vi "HDF5_Test2.vi"   [LabVIEW 2018]
uses:
  <vilib>/addons/h5labview2/base/H5Equery.vi
  HDF5/lib_path_mod_20200519.vi
  HDF5/HDF5_ToneInfoClust.ctl
  <vilib>/addons/h5labview2/attrib/H5Awrite.llb/H5Awrite.xnode
  <vilib>/addons/h5labview2/base/hid_t_renamed.ctl
  <vilib>/addons/h5labview2/file/H5F.lvlib
  <vilib>/addons/h5labview2/file/H5Fmode.ctl
  Controls/Clusts/LogLoopClust.ctl
  Controls/ToneInfoClust.ctl
  Controls/Clusts/ChannelToneData.ctl
  Controls/Enums/TargetNumber.ctl
  <vilib>/addons/h5labview2/group/H5G.lvlib
  <vilib>/addons/h5labview2/dataset/H5D.lvlib
  HDF5/HDF5_Tone_refs.ctl
  HDF5/HDF5_Complex_Refs.ctl
  HDF5/HDF5_ADAM_Refs.ctl
  HDF5/HDF5_Filter_refs.ctl
  HDF5/HDF5_AI_refs.ctl
  Controls/PathsCluster.ctl
  Controls/Enums/ScaleMeasure.ctl
  Controls/Clusts/FPGA_Scale.ctl
  Controls/Clusts/FreqShift.ctl
  Controls/Clusts/FP_UserTargetConfig.ctl
  Controls/Clusts/FrontPanel_UserConfig.ctl
  Controls/Clusts/UserConfig.ctl
  Controls/Clusts/Config_Clust.ctl
  Controls/Clusts/WeatherRefs.ctl
  HDF5/UPS_refs.ctl
  HDF5/HDF5_Health_Refs.ctl
  HDF5/HDF5_Disdrometer_Refs.ctl
  HDF5/HDF5_Validty_refs.ctl
  HDF5/TC_Tone_refs.ctl
  HDF5/HDF5_Noise_refs.ctl
  Controls/Clusts/ToneGroupRefsClust.ctl
  Controls/Clusts/TimeDomainData.ctl
  HDF5/HDF5_ADAM_Data.ctl
  Controls/Clusts/TE_Data_Clust.ctl
  Controls/Clusts/WeatherDataClust.ctl
  Disdrometer/Disdrometer_Status_Cluster.ctl
  HDF5/DisdromterSummaryData.ctl
  HDF5/DisdrometerData.ctl
  HDF5/HDF5_NoiseInfoClust.ctl
  Controls/Clusts/AI_Clust.ctl
  HDF5/TC_Data_Structure.ctl
  Controls/Clusts/ToneLogBuffered.ctl
  Controls/Clusts/LogDataClust.ctl
  Controls/Clusts/HDF5_File_Refs.ctl
  Controls/RadioButtons/FilterEnableRadio.ctl
  Controls/Clusts/Inclinometer_User_Cfg.ctl
  Controls/Clusts/AlarmThresh_OneChan.ctl
  Controls/Clusts/AlarmSettingsClust.ctl
  Controls/Clusts/ErrorStatus.ctl
  Controls/Clusts/ValidityWeatherClust.ctl
  Controls/Clusts/SaturationMonitorBuffer.ctl
  Controls/Clusts/HDF5_10HzRefs.ctl
  Controls/Clusts/Saturation_Status_Clust.ctl
  <vilib>/addons/h5labview2/base/hid_t.ctl
  Controls/Clusts/DigOutClust.ctl
types:
  T1 = typedef "HDF5_ToneInfoClust.ctl" = cluster{"Timestring":string, "Timestamp":dbl, "MaxValue":dbl, "PeakLoc":dbl, "df":dbl}
  T2 = typedef "LogLoopClust.ctl" = cluster{"base path":path, "PathNow1":path, "PathNow2":path, "DateNow":string, "NAS path":path, "LogFiltStage":bool, "Config":T3, "HDFRefs1":T14, "HDFRefs2":T14, "LogData":T29, "AlarmCfg":T43, "DO":bool[], "AllAlarms":T45[], "Alarm Status":T46, "SaturationStatus":T47, "WeatherStatus":bool[], "10HzRefs":T48}
  T3 = typedef "Config_Clust.ctl" = cluster{"UsrCfg":T4, "FP_User":T6}
  T4 = typedef "UserConfig.ctl" = cluster{"Paths":T5, "SampleRate":dbl}
  T5 = typedef "PathsCluster.ctl" = cluster{"CfgFile":path, "LogFolder":path, "LogFile":path, "NAS path":path, "ThreshFile":path, "RedunFolder":path}
  T6 = typedef "FrontPanel_UserConfig.ctl" = cluster{"#NoiseSums":u32, "Max_df":u32, "AvgAvg":bool, "#Avg":u16, "AutoCenter":bool, "Inclin":T7, "1":T8, "2":T8, "3":T8, "4":T8, "Target to Probe":T13, "SNR_Thresh":dbl, "Paths":T5, "Connex_Location":string, "SimulateFPGA":bool}
  T7 = typedef "Inclinometer_User_Cfg.ctl" = cluster{"Vmin":dbl, "Vmax":dbl, "Angle_min":dbl, "Angle_max":dbl, "Offset":dbl, "Pos_Neg":bool}
  T8 = typedef "FP_UserTargetConfig.ctl" = cluster{"Cal_":T9, "Beac":T9, "Scale":T10, "Offset":fxp<+/-,16,16>, "Scale_Noise":fxp<+/-,30,30>, "Scale_Step1":fxp<+/-,17,17>, "Scale_In_RT":ext, "ScaleMeas":fxp<+/-,16,1>, "FreqsToRemove":i32[], "Width":i32[], "ScaleMeasEnum":T11, "FilterEnab":T12}
  T9 = typedef "FreqShift.ctl" = cluster{"Fine":dbl, "Coarse_":dbl}
  T10 = typedef "FPGA_Scale.ctl" = cluster{"Step4":fxp<+/-,23,23>, "Step5":fxp<+/-,23,23>, "Step6":fxp<+/-,23,23>, "Step7":fxp<+/-,23,23>}
  T11 = typedef "ScaleMeasure.ctl" = enum16{"1", "10", "50", "42"}
  T12 = typedef "FilterEnableRadio.ctl" = enum32{"None", "Step 1", "Frequency Shift", "Step 4", "Step 5", "Step 6", "Step 7"}
  T13 = typedef "TargetNumber.ctl" = enum16{"1", "2", "3", "4"}
  T14 = typedef "HDF5_File_Refs.ctl" = cluster{"File":T15, "ToneRefs":T16[], "NoiseRefs":T18[], "TC_Refs":T19, "ValidRefs":T20, "DisdromRefs":T21, "TE_Refs":T22, "UPS_Refs_Deprecated":T23, "Weath_Refs":T24, "AI_Refs":T25, "Filter_Refs":T26, "ADAM_Refs":T27, "Complex":T28[]}
  T15 = typedef "hid_t.ctl" = i32
  T16 = typedef "ToneGroupRefsClust.ctl" = cluster{"Group_ref":T15, "Cal":T17, "Beac":T17, "CalZoom_dSet":T15, "BeacZoom_dSet":T15}
  T17 = typedef "HDF5_Tone_refs.ctl" = cluster{"TimeString_dset":T15, "TImeStamp_dset":T15, "SNR_dset":T15, "MaxValue_dset":T15, "PeakLoc_dset":T15, "df_dset":T15, "Phase_dset":T15, "DeltaPhase_dset":T15, "Downshift_dset":T15}
  T18 = typedef "HDF5_Noise_refs.ctl" = cluster{"Group_ref":T15, "TimeString_dset":T15, "TimeStamp_dset":T15, "df_dset":T15, "sum_dset":T15, "SumdSpectrum_dset":T15}
  T19 = typedef "TC_Tone_refs.ctl" = cluster{"Group_ref":T15, "TimeString_dset":T15, "TimeStamp_dset":T15, "TC0_LP1_Hi":T15, "TC1_LP1_MidHi":T15, "TC2_LP1_Mid":T15, "TC3_LP1_LoMid":T15, "TC4_LP1_Lo":T15, "TC5_LP2_Hi":T15, "TC6_LP2_MidHi":T15, "TC7_LP2_Mid":T15, "TC8_LP2_LoMid":T15, "TC9_LP2_Lo":T15, "TC10_HVAC_Cond_In":T15, "TC11_HVAC_Cond_Out":T15, "TC12_Gen_Exhaust":T15, "TC13_Tamb_Inter":T15}
  T20 = typedef "HDF5_Validty_refs.ctl" = cluster{"Group_ref":T15, "Weath_Valid_dset":T15, "Disdr_Valid_dset":T15, "Saturat_dset":T15, "Alarm_Valid_dset":T15, "Time_Valid_dset":T15, "Time_AlarmChange_dset":T15, "Alarm_Source_dset":T15}
  T21 = typedef "HDF5_Disdrometer_Refs.ctl" = cluster{"BasicGroup_ref":T15, "TimeStamp_dset":T15, "TotalRainRate_dset":T15, "Liquid_dset":T15, "Solid_dset":T15, "TotalRain_dset":T15, "Visibility_dset":T15, "RadarReflect_dset":T15, "MaxDiam_dset":T15, "MeasdParticles_dset":T15, "ParticlMinSpeed_dset":T15, "ParticlMaxSpeed_dset":T15, "ParticlMinDiam_dset":T15, "NonHydrParticls_dset":T15, "NonHydrVolum_dset":T15, "UnknownParticls_dset":T15, "UnknownVolum_dset":T15, "HydromType_dset":T15, "SpectGroup_ref":T15, "Spectrum_dset":T15, "Status_dset_deprecated":T15}
  T22 = typedef "HDF5_Health_Refs.ctl" = cluster{"Group_ref":T15, "TE_Temp1_dset":T15, "TE_Outp1_dset":T15, "TE_Temp2_dset":T15, "TE_Outp2_dset":T15, "TE_Temp3_dset":T15, "TE_Outp3_dset":T15, "TimeStamp":T15}
  T23 = typedef "UPS_refs.ctl" = cluster{"Group_ref":T15, "TimeString_dset":T15, "TimeStamp_dset":T15, "V_dset":T15, "A_dset":T15, "Hz_dset":T15, "W_dset":T15, "%_dset":T15}
  T24 = typedef "WeatherRefs.ctl" = cluster{"Group_ref":T15, "TimeString_dset":T15, "TimeStamp_dset ":T15, "WindSpd_dset":T15, "WindGusts_dset":T15, "WindDir_dset":T15, "WindDirSTD_dset":T15, "Temp_dset":T15, "Humidity_dset":T15, "Pressure_dset":T15, "RainRate_dset":T15, "RainFall_dset":T15}
  T25 = typedef "HDF5_AI_refs.ctl" = cluster{"Group_ref":T15, "TimeString_dset":T15, "TimeStamp_dset":T15, "AI0_dset":T15, "AI1_dset":T15, "AI2_dset":T15, "AI3_dset":T15, "AI4_dset":T15, "AI5_dset":T15, "AI6_dset":T15, "AI16_dset":T15, "AI17_dset":T15, "AI18_dset":T15, "AzStdDev_dset":T15, "AI19_dset":T15, "ElStdDev_dset":T15, "BlowerPwr_dset":T15}
  T26 = typedef "HDF5_Filter_refs.ctl" = cluster{"Filter_Group_ref":T15, "TimeStamp_dset":T15, "Filter_dset":T15}
  T27 = typedef "HDF5_ADAM_Refs.ctl" = cluster{"Group_ref":T15, "ADAM_CoPol_dset":T15, "ADAM_XPol_dset":T15, "ADAM_Noise_dset":T15, "ADAM_CalBox_dset":T15, "TimeStamp":T15}
  T28 = typedef "HDF5_Complex_Refs.ctl" = cluster{"Group_ref":T15, "TImeStamp_dset":T15, "PwrSpect_dset":T15, "ISpect_dset":T15, "QSpect_dset":T15}
  T29 = typedef "LogDataClust.ctl" = cluster{"Tone":T30[], "TCData":T32, "AI":T33, "NoiseTrace":cluster{"Target":T13, "NoiseTrace":dbl[]}[], "NoiseInfo":cluster{"Target":T13, "HDF5_NoiseInfo":T34}[], "Disdrom":T35[], "Weath":T38[], "TE":T40, "ADAM":T41, "TimeDomain":T42[]}
  T30 = typedef "ToneLogBuffered.ctl" = cluster{"Count":i32, "CalVal":sgl[], "CalLoc":sgl[], "BeacVal":sgl[], "BeacLoc":sgl[], "BeacShift":sgl[], "Enum":T13, "df":dbl, "PwrSpectr":sgl[][], "ISpectr":sgl[][], "QSpectr":sgl[][], "Time":timestamp[], "SNR":sgl[], "AboveThresh":bool[], "10Hz_PeakVal":dbl[], "Phase":sgl[], "DeltaPhase":dbl[], "Saturat":T31}
  T31 = typedef "SaturationMonitorBuffer.ctl" = cluster{"Meas":bool[], "Stage1":bool[], "Stage4":bool[], "Stage5":bool[], "Stage6":bool[], "Stage7":bool[]}
  T32 = typedef "TC_Data_Structure.ctl" = cluster{"TimeStamp":dbl, "TimeString":string, "TC0_LP1_Hi":dbl, "TC1_LP1_MidHi":dbl, "TC2_LP1_Mid":dbl, "TC3_LP1_LoMid":dbl, "TC4_LP1_Lo":dbl, "TC5_LP2_Hi":dbl, "TC6_LP2_MidHi":dbl, "TC7_LP2_Mid":dbl, "TC8_LP2_LoMid":dbl, "TC9_LP2_Lo":dbl, "TC10_HVAC_Cond_In":dbl, "TC11_HVAC_Cond_Out":dbl, "TC12_Gen_Exhaust":dbl, "TC13_Unused":dbl, "TC14_Unused":dbl, "TC15_Unused":dbl, "TC16_Unused":dbl, "TC17_Unused":dbl, "TC18_Unused":dbl, "TC19_Unused":dbl, "TC20_Unused":dbl, "TC21_Unused":dbl, "TC22_Unused":dbl, "TC23_Unused":dbl, "TC24_Unused":dbl, "TC25_Unused":dbl, "TC26_Unused":dbl, "TC27_Unused":dbl, "TC28_Unused":dbl, "TC29_Unused":dbl, "TC30_Unused":dbl, "TC31_Unused":dbl}
  T33 = typedef "AI_Clust.ctl" = cluster{"TimeString":string, "Time Stamp":dbl, "AI0_Unused":dbl, "AI1_-5V":dbl, "AI2_+5V":dbl, "AI3_+6V":dbl, "AI4_+12V":dbl, "AI5_+15V":dbl, "AI6_+28V":dbl, "AI7_Unused":dbl, "Ai16_72GHz_CalPower":dbl, "Ai17_84GHz_CalPower":dbl, "Ai18_InclinAz":dbl, "Ai19_InclinEl":dbl, "Ai20_BlowerPwr":dbl, "Ai21_Unused":dbl, "Ai22_Unused":dbl, "Ai23_Unused":dbl, "InclinA_StdDev":dbl, "InclinB_StdDev":dbl, "InclinAz_Unfilt":dbl, "InclinEl_Unfilt":dbl}
  T34 = typedef "HDF5_NoiseInfoClust.ctl" = cluster{"Timestring":string, "Timestamp":dbl, "df":dbl, "Sum":dbl}
  T35 = typedef "DisdrometerData.ctl" = cluster{"Spectrum Data":i16[], "DisdromSummary":T36, "Status":T37}
  T36 = typedef "DisdromterSummaryData.ctl" = cluster{"current time":dbl, "Timestamp":dbl, "Total Rain Rate":dbl, "Liquid Rain Rate":dbl, "Solid Rain Rate":dbl, "Total Rainfall":dbl, "Visibility":dbl, "Radar Reflectivity":dbl, "Max Diameter Hail":dbl, "Measured Particles":i16, "Particle Min Speed":i16, "Particle Max Speed":i16, "Particle Min Diam":i16, "NonHydr Particles":i16, "NonHydr Volume":dbl, "Unkn Particles":i16, "Unkn Volume":dbl, "HydroType":i8}
  T37 = typedef "Disdrometer_Status_Cluster.ctl" = cluster{"Laser":bool, "Signal":bool, "LaserTemp_Analog":bool, "LaserTemp_Digital":bool, "LaserCurrent_Analog":bool, "LaserCurrent_Digital":bool, "SensorSupply":bool, "HeatLaserHead":bool, "HeatReceiverHead":bool, "TempSensor":bool, "HeatSupply":bool, "HeatHousing":bool, "HeatHeads":bool, "HeatCarriers":bool, "OutputLaserPower":bool, "Checksum":bool, "StatusInt":u16}
  T38 = typedef "WeatherDataClust.ctl" = cluster{"TimeString":string, "Timestamp":dbl, "Wind Speed":sgl, "Wind Gusts":sgl, "Wind Dir":sgl, "Wind Dir STD":sgl, "Temperature":sgl, "Humidity":sgl, "Pressure":sgl, "Rain Rate":i16, "Rain Fall":sgl, "Status":T39}
  T39 = typedef "ValidityWeatherClust.ctl" = cluster{"Temp_OutOfBounds":bool, "Temp_IncrSTD":bool, "Temp_Oth":bool, "BarPress_OutOfBounds":bool, "BarPress_IncrSTD":bool, "BarPress_Change":bool, "BarPress_Other":bool, "Humid_OutOfBounds":bool, "Humid_IncrSTD":bool, "Humid_Other":bool, "Wind__Spd_OutOfBounds":bool, "Wind_Dir_OutOfBounds":bool, "RainBuck_OutOfBounds":bool, "RainBuck_Disdrom":bool, "Disdrom_RainBuck":bool, "Placeholder":bool}
  T40 = typedef "TE_Data_Clust.ctl" = cluster{"TimeString":string, "TimeStamp":dbl, "Temp":dbl, "Output":dbl, "Temp 2":dbl, "Output 2":dbl, "Temp 3":dbl, "Output 3":dbl}
  T41 = typedef "HDF5_ADAM_Data.ctl" = cluster{"Timestamp":dbl, "Time string":string, "Fault 1":bool, "Fault 2":bool, "Fault 3":bool, "Fault 4":bool, "Fault 5":bool, "Fault 6":bool, "Value 1":dbl, "Value 2":dbl, "Value 3":dbl, "Value 4":dbl, "Value 5":dbl, "Value 6":dbl}
  T42 = typedef "TimeDomainData.ctl" = cluster{"CalTimeVal":dbl[], "CalTimeCount":u32[], "Enum":T13}
  T43 = typedef "AlarmSettingsClust.ctl" = cluster{"TC13":T44, "AI1":T44, "AI2":T44, "AI3":T44, "AI4":T44, "AI5":T44, "AI6":T44, "AI18":T44, "AI19":T44, "TE1":T44, "TE2":T44, "TE3":T44, "ADAM1":T44, "ADAM2":T44, "ADAM3":T44, "ADAM4":T44, "72CoBeacFreq":T44, "72CoCalFreq":T44, "84CoBeacFreq":T44, "84CoCalFreq":T44, "72Co_CalTonePwr":T44, "72X_CalTonePwr":T44, "84Co_CalTonePwr":T44, "84X_CalTonePwr":T44}
  T44 = typedef "AlarmThresh_OneChan.ctl" = cluster{"Enbl":bool, "ErrsAndWarns":cluster{dbl, dbl, dbl, dbl}}
  T45 = typedef "ErrorStatus.ctl" = cluster{"RX?":bool, "Warn":bool, "Error":bool, "Enabl":bool, "Source":string}
  T46 = typedef "DigOutClust.ctl" = cluster{"Green":bool, "Rx_Yell":bool, "Cx_Yell":bool, "Red":bool, "Source":string}
  T47 = typedef "Saturation_Status_Clust.ctl" = cluster{"84":bool[], "72":bool[]}
  T48 = typedef "HDF5_10HzRefs.ctl" = cluster{"72Co_dset":T15, "84Co_dset":T15, "FileRef":T15}
  T49 = typedef "H5F.lvlib/H5Fmode.ctl" = enum16{"read-only", "read-write", "overwrite", "create new", "open or create"}
  T50 = typedef "ChannelToneData.ctl" = cluster{"LastPk":dbl, "Shift_":dbl, "Pk_PreShift":dbl, "Peak_ToFPGA":dbl, "MaxValue":dbl, "MaxIndex":i32, "Tone":T51, "TimeDomainI":ext[], "TimeDomainQ":ext[], "PwrSpectrum":dbl[], "RunningAvgFreq":dbl, "PhaseSpect":dbl[], "RealSpect":dbl[], "ImagSpect":dbl[]}
  T51 = typedef "ToneInfoClust.ctl" = cluster{"PeakLoc":dbl, "df_":dbl, "ZoomPwr":dbl[], "ZoomPhase":dbl[]}
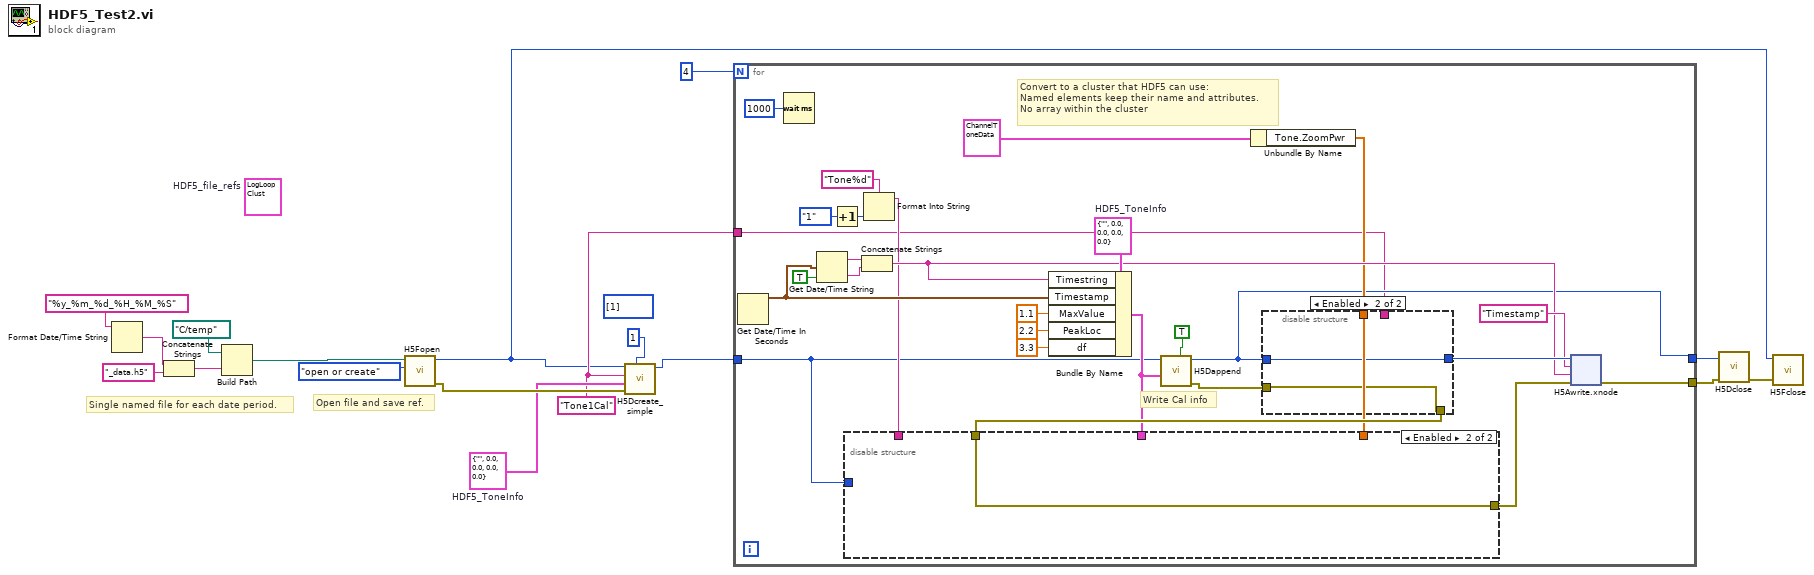
[diagram p0: block diagram]
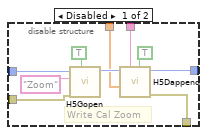
[diagram p2: hidden frame]
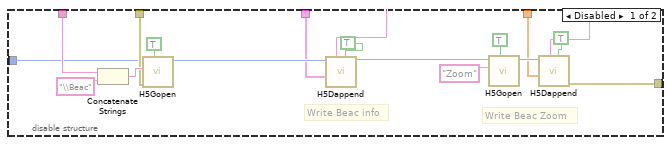
[diagram p3: hidden frame]
diagram:
  (unwired) u64[] [1] ("chunk size")
  w8 = T1 {"Timestring"="", "Timestamp"=0.0, "MaxValue"=0.0, "PeakLoc"=0.0, "df"=0.0}  # HDF5_ToneInfo
  w3 = "Tone1Cal" ("name")
  (unwired) T2 {"base path"=path "", "PathNow1"=path "", "PathNow2"=path "", "DateNow"="", "NAS path"=path "", "LogFiltStage"=FALSE, "Config"={"UsrCfg"={"Paths"={"CfgFile"=path "", "LogFolder"=path "", "LogFile"=path "", "NAS path"=path "", "ThreshFile"=path "", "RedunFolder"=path ""}, "SampleRate"=0.0}, "FP_User"={"#NoiseSums"=0, "Max_df"=0, "AvgAvg"=FALSE, "#Avg"=0, "AutoCenter"=FALSE, "Inclin"={"Vmin"=0.0, "Vmax"=0.0, "Angle_min"=0.0, "Angle_max"=0.0, "Offset"=0.0, "Pos_Neg"=FALSE}, "1"={"Cal_"={"Fine"=0.0, "Coarse_"=0.0}, "Beac"={"Fine"=0.0, "Coarse_"=0.0}, "Scale"={"Step4"=0.0, "Step5"=0.0, "Step6"=0.0, "Step7"=0.0}, "Offset"=0.0, "Scale_Noise"=0.0, "Scale_Step1"=0.0, "Scale_In_RT"=0.0, "ScaleMeas"=0.0, "FreqsToRemove"=[], "Width"=[], "ScaleMeasEnum"=enum."1", "FilterEnab"=enum."None"}, "2"={"Cal_"={"Fine"=0.0, "Coarse_"=0.0}, "Beac"={"Fine"=0.0, "Coarse_"=0.0}, "Scale"={"Step4"=0.0, "Step5"=0.0, "Step6"=0.0, "Step7"=0.0}, "Offset"=0.0, "Scale_Noise"=0.0, "Scale_Step1"=0.0, "Scale_In_RT"=0.0, "ScaleMeas"=0.0, "FreqsToRemove"=[], "Width"=[], "ScaleMeasEnum"=enum."1", "FilterEnab"=enum."None"}, "3"={"Cal_"={"Fine"=0.0, "Coarse_"=0.0}, "Beac"={"Fine"=0.0, "Coarse_"=0.0}, "Scale"={"Step4"=0.0, "Step5"=0.0, "Step6"=0.0, "Step7"=0.0}, "Offset"=0.0, "Scale_Noise"=0.0, "Scale_Step1"=0.0, "Scale_In_RT"=0.0, "ScaleMeas"=0.0, "FreqsToRemove"=[], "Width"=[], "ScaleMeasEnum"=enum."1", "FilterEnab"=enum."None"}, "4"={"Cal_"={"Fine"=0.0, "Coarse_"=0.0}, "Beac"={"Fine"=0.0, "Coarse_"=0.0}, "Scale"={"Step4"=0.0, "Step5"=0.0, "Step6"=0.0, "Step7"=0.0}, "Offset"=0.0, "Scale_Noise"=0.0, "Scale_Step1"=0.0, "Scale_In_RT"=0.0, "ScaleMeas"=0.0, "FreqsToRemove"=[], "Width"=[], "ScaleMeasEnum"=enum."1", "FilterEnab"=enum."None"}, "Target to Probe"=enum."1", "SNR_Thresh"=0.0, "Paths"={"CfgFile"=path "", "LogFolder"=path "", "LogFile"=path "", "NAS path"=path "", "ThreshFile"=path "", "RedunFolder"=path ""}, "Connex_Location"="", "SimulateFPGA"=FALSE}}, "HDFRefs1"={"File"=0, "ToneRefs"=[], "NoiseRefs"=[], "TC_Refs"={"Group_ref"=0, "TimeString_dset"=0, "TimeStamp_dset"=0, "TC0_LP1_Hi"=0, "TC1_LP1_MidHi"=0, "TC2_LP1_Mid"=0, "TC3_LP1_LoMid"=0, "TC4_LP1_Lo"=0, "TC5_LP2_Hi"=0, "TC6_LP2_MidHi"=0, "TC7_LP2_Mid"=0, "TC8_LP2_LoMid"=0, "TC9_LP2_Lo"=0, "TC10_HVAC_Cond_In"=0, "TC11_HVAC_Cond_Out"=0, "TC12_Gen_Exhaust"=0, "TC13_Tamb_Inter"=0}, "ValidRefs"={"Group_ref"=0, "Weath_Valid_dset"=0, "Disdr_Valid_dset"=0, "Saturat_dset"=0, "Alarm_Valid_dset"=0, "Time_Valid_dset"=0, "Time_AlarmChange_dset"=0, "Alarm_Source_dset"=0}, "DisdromRefs"={"BasicGroup_ref"=0, "TimeStamp_dset"=0, "TotalRainRate_dset"=0, "Liquid_dset"=0, "Solid_dset"=0, "TotalRain_dset"=0, "Visibility_dset"=0, "RadarReflect_dset"=0, "MaxDiam_dset"=0, "MeasdParticles_dset"=0, "ParticlMinSpeed_dset"=0, "ParticlMaxSpeed_dset"=0, "ParticlMinDiam_dset"=0, "NonHydrParticls_dset"=0, "NonHydrVolum_dset"=0, "UnknownParticls_dset"=0, "UnknownVolum_dset"=0, "HydromType_dset"=0, "SpectGroup_ref"=0, "Spectrum_dset"=0, "Status_dset_deprecated"=0}, "TE_Refs"={"Group_ref"=0, "TE_Temp1_dset"=0, "TE_Outp1_dset"=0, "TE_Temp2_dset"=0, "TE_Outp2_dset"=0, "TE_Temp3_dset"=0, "TE_Outp3_dset"=0, "TimeStamp"=0}, "UPS_Refs_Deprecated"={"Group_ref"=0, "TimeString_dset"=0, "TimeStamp_dset"=0, "V_dset"=0, "A_dset"=0, "Hz_dset"=0, "W_dset"=0, "%_dset"=0}, "Weath_Refs"={"Group_ref"=0, "TimeString_dset"=0, "TimeStamp_dset "=0, "WindSpd_dset"=0, "WindGusts_dset"=0, "WindDir_dset"=0, "WindDirSTD_dset"=0, "Temp_dset"=0, "Humidity_dset"=0, "Pressure_dset"=0, "RainRate_dset"=0, "RainFall_dset"=0}, "AI_Refs"={"Group_ref"=0, "TimeString_dset"=0, "TimeStamp_dset"=0, "AI0_dset"=0, "AI1_dset"=0, "AI2_dset"=0, "AI3_dset"=0, "AI4_dset"=0, "AI5_dset"=0, "AI6_dset"=0, "AI16_dset"=0, "AI17_dset"=0, "AI18_dset"=0, "AzStdDev_dset"=0, "AI19_dset"=0, "ElStdDev_dset"=0, "BlowerPwr_dset"=0}, "Filter_Refs"={"Filter_Group_ref"=0, "TimeStamp_dset"=0, "Filter_dset"=0}, "ADAM_Refs"={"Group_ref"=0, "ADAM_CoPol_dset"=0, "ADAM_XPol_dset"=0, "ADAM_Noise_dset"=0, "ADAM_CalBox_dset"=0, "TimeStamp"=0}, "Complex"=[]}, "HDFRefs2"={"File"=0, "ToneRefs"=[], "NoiseRefs"=[], "TC_Refs"={"Group_ref"=0, "TimeString_dset"=0, "TimeStamp_dset"=0, "TC0_LP1_Hi"=0, "TC1_LP1_MidHi"=0, "TC2_LP1_Mid"=0, "TC3_LP1_LoMid"=0, "TC4_LP1_Lo"=0, "TC5_LP2_Hi"=0, "TC6_LP2_MidHi"=0, "TC7_LP2_Mid"=0, "TC8_LP2_LoMid"=0, "TC9_LP2_Lo"=0, "TC10_HVAC_Cond_In"=0, "TC11_HVAC_Cond_Out"=0, "TC12_Gen_Exhaust"=0, "TC13_Tamb_Inter"=0}, "ValidRefs"={"Group_ref"=0, "Weath_Valid_dset"=0, "Disdr_Valid_dset"=0, "Saturat_dset"=0, "Alarm_Valid_dset"=0, "Time_Valid_dset"=0, "Time_AlarmChange_dset"=0, "Alarm_Source_dset"=0}, "DisdromRefs"={"BasicGroup_ref"=0, "TimeStamp_dset"=0, "TotalRainRate_dset"=0, "Liquid_dset"=0, "Solid_dset"=0, "TotalRain_dset"=0, "Visibility_dset"=0, "RadarReflect_dset"=0, "MaxDiam_dset"=0, "MeasdParticles_dset"=0, "ParticlMinSpeed_dset"=0, "ParticlMaxSpeed_dset"=0, "ParticlMinDiam_dset"=0, "NonHydrParticls_dset"=0, "NonHydrVolum_dset"=0, "UnknownParticls_dset"=0, "UnknownVolum_dset"=0, "HydromType_dset"=0, "SpectGroup_ref"=0, "Spectrum_dset"=0, "Status_dset_deprecated"=0}, "TE_Refs"={"Group_ref"=0, "TE_Temp1_dset"=0, "TE_Outp1_dset"=0, "TE_Temp2_dset"=0, "TE_Outp2_dset"=0, "TE_Temp3_dset"=0, "TE_Outp3_dset"=0, "TimeStamp"=0}, "UPS_Refs_Deprecated"={"Group_ref"=0, "TimeString_dset"=0, "TimeStamp_dset"=0, "V_dset"=0, "A_dset"=0, "Hz_dset"=0, "W_dset"=0, "%_dset"=0}, "Weath_Refs"={"Group_ref"=0, "TimeString_dset"=0, "TimeStamp_dset "=0, "WindSpd_dset"=0, "WindGusts_dset"=0, "WindDir_dset"=0, "WindDirSTD_dset"=0, "Temp_dset"=0, "Humidity_dset"=0, "Pressure_dset"=0, "RainRate_dset"=0, "RainFall_dset"=0}, "AI_Refs"={"Group_ref"=0, "TimeString_dset"=0, "TimeStamp_dset"=0, "AI0_dset"=0, "AI1_dset"=0, "AI2_dset"=0, "AI3_dset"=0, "AI4_dset"=0, "AI5_dset"=0, "AI6_dset"=0, "AI16_dset"=0, "AI17_dset"=0, "AI18_dset"=0, "AzStdDev_dset"=0, "AI19_dset"=0, "ElStdDev_dset"=0, "BlowerPwr_dset"=0}, "Filter_Refs"={"Filter_Group_ref"=0, "TimeStamp_dset"=0, "Filter_dset"=0}, "ADAM_Refs"={"Group_ref"=0, "ADAM_CoPol_dset"=0, "ADAM_XPol_dset"=0, "ADAM_Noise_dset"=0, "ADAM_CalBox_dset"=0, "TimeStamp"=0}, "Complex"=[]}, "LogData"={"Tone"=[], "TCData"={"TimeStamp"=0.0, "TimeString"="", "TC0_LP1_Hi"=0.0, "TC1_LP1_MidHi"=0.0, "TC2_LP1_Mid"=0.0, "TC3_LP1_LoMid"=0.0, "TC4_LP1_Lo"=0.0, "TC5_LP2_Hi"=0.0, "TC6_LP2_MidHi"=0.0, "TC7_LP2_Mid"=0.0, "TC8_LP2_LoMid"=0.0, "TC9_LP2_Lo"=0.0, "TC10_HVAC_Cond_In"=0.0, "TC11_HVAC_Cond_Out"=0.0, "TC12_Gen_Exhaust"=0.0, "TC13_Unused"=0.0, "TC14_Unused"=0.0, "TC15_Unused"=0.0, "TC16_Unused"=0.0, "TC17_Unused"=0.0, "TC18_Unused"=0.0, "TC19_Unused"=0.0, "TC20_Unused"=0.0, "TC21_Unused"=0.0, "TC22_Unused"=0.0, "TC23_Unused"=0.0, "TC24_Unused"=0.0, "TC25_Unused"=0.0, "TC26_Unused"=0.0, "TC27_Unused"=0.0, "TC28_Unused"=0.0, "TC29_Unused"=0.0, "TC30_Unused"=0.0, "TC31_Unused"=0.0}, "AI"={"TimeString"="", "Time Stamp"=0.0, "AI0_Unused"=0.0, "AI1_-5V"=0.0, "AI2_+5V"=0.0, "AI3_+6V"=0.0, "AI4_+12V"=0.0, "AI5_+15V"=0.0, "AI6_+28V"=0.0, "AI7_Unused"=0.0, "Ai16_72GHz_CalPower"=0.0, "Ai17_84GHz_CalPower"=0.0, "Ai18_InclinAz"=0.0, "Ai19_InclinEl"=0.0, "Ai20_BlowerPwr"=0.0, "Ai21_Unused"=0.0, "Ai22_Unused"=0.0, "Ai23_Unused"=0.0, "InclinA_StdDev"=0.0, "InclinB_StdDev"=0.0, "InclinAz_Unfilt"=0.0, "InclinEl_Unfilt"=0.0}, "NoiseTrace"=[], "NoiseInfo"=[], "Disdrom"=[], "Weath"=[], "TE"={"TimeString"="", "TimeStamp"=0.0, "Temp"=0.0, "Output"=0.0, "Temp 2"=0.0, "Output 2"=0.0, "Temp 3"=0.0, "Output 3"=0.0}, "ADAM"={"Timestamp"=0.0, "Time string"="", "Fault 1"=FALSE, "Fault 2"=FALSE, "Fault 3"=FALSE, "Fault 4"=FALSE, "Fault 5"=FALSE, "Fault 6"=FALSE, "Value 1"=0.0, "Value 2"=0.0, "Value 3"=0.0, "Value 4"=0.0, "Value 5"=0.0, "Value 6"=0.0}, "TimeDomain"=[]}, "AlarmCfg"={"TC13"={"Enbl"=FALSE, "ErrsAndWarns"={0.0, 0.0, 0.0, 0.0}}, "AI1"={"Enbl"=FALSE, "ErrsAndWarns"={0.0, 0.0, 0.0, 0.0}}, "AI2"={"Enbl"=FALSE, "ErrsAndWarns"={0.0, 0.0, 0.0, 0.0}}, "AI3"={"Enbl"=FALSE, "ErrsAndWarns"={0.0, 0.0, 0.0, 0.0}}, "AI4"={"Enbl"=FALSE, "ErrsAndWarns"={0.0, 0.0, 0.0, 0.0}}, "AI5"={"Enbl"=FALSE, "ErrsAndWarns"={0.0, 0.0, 0.0, 0.0}}, "AI6"={"Enbl"=FALSE, "ErrsAndWarns"={0.0, 0.0, 0.0, 0.0}}, "AI18"={"Enbl"=FALSE, "ErrsAndWarns"={0.0, 0.0, 0.0, 0.0}}, "AI19"={"Enbl"=FALSE, "ErrsAndWarns"={0.0, 0.0, 0.0, 0.0}}, "TE1"={"Enbl"=FALSE, "ErrsAndWarns"={0.0, 0.0, 0.0, 0.0}}, "TE2"={"Enbl"=FALSE, "ErrsAndWarns"={0.0, 0.0, 0.0, 0.0}}, "TE3"={"Enbl"=FALSE, "ErrsAndWarns"={0.0, 0.0, 0.0, 0.0}}, "ADAM1"={"Enbl"=FALSE, "ErrsAndWarns"={0.0, 0.0, 0.0, 0.0}}, "ADAM2"={"Enbl"=FALSE, "ErrsAndWarns"={0.0, 0.0, 0.0, 0.0}}, "ADAM3"={"Enbl"=FALSE, "ErrsAndWarns"={0.0, 0.0, 0.0, 0.0}}, "ADAM4"={"Enbl"=FALSE, "ErrsAndWarns"={0.0, 0.0, 0.0, 0.0}}, "72CoBeacFreq"={"Enbl"=FALSE, "ErrsAndWarns"={0.0, 0.0, 0.0, 0.0}}, "72CoCalFreq"={"Enbl"=FALSE, "ErrsAndWarns"={0.0, 0.0, 0.0, 0.0}}, "84CoBeacFreq"={"Enbl"=FALSE, "ErrsAndWarns"={0.0, 0.0, 0.0, 0.0}}, "84CoCalFreq"={"Enbl"=FALSE, "ErrsAndWarns"={0.0, 0.0, 0.0, 0.0}}, "72Co_CalTonePwr"={"Enbl"=FALSE, "ErrsAndWarns"={0.0, 0.0, 0.0, 0.0}}, "72X_CalTonePwr"={"Enbl"=FALSE, "ErrsAndWarns"={0.0, 0.0, 0.0, 0.0}}, "84Co_CalTonePwr"={"Enbl"=FALSE, "ErrsAndWarns"={0.0, 0.0, 0.0, 0.0}}, "84X_CalTonePwr"={"Enbl"=FALSE, "ErrsAndWarns"={0.0, 0.0, 0.0, 0.0}}}, "DO"=[], "AllAlarms"=[], "Alarm Status"={"Green"=FALSE, "Rx_Yell"=FALSE, "Cx_Yell"=FALSE, "Red"=FALSE, "Source"=""}, "SaturationStatus"={"84"=[], "72"=[]}, "WeatherStatus"=[], "10HzRefs"={"72Co_dset"=0, "84Co_dset"=0, "FileRef"=0}}  # HDF5_file_refs
  # "Open file and save ref."
  # "Single named file for each date period."
  n1 = Format Date/Time String(time format string (%c)="%y_%m_%d_%H_%M_%S") -> (date/time string=w12:string)  [unwired: 2 in]
  n2 = Concatenate Strings(w12, "_data.h5" ("string")) -> (w16:string)
  n3 = Build Path(base path=path "C:/temp", name or relative path=w16) -> (appended path=w14:path)
  n4 = call <vilib>:"H5Fopen.vi"("mode (read-only)"=H5Fmode."open or create", "path"=w14) -> ("error out"=w9:errorcluster, "ref out"=w2:T15)  [unwired: 8 in]
  n5 = call <vilib>:"H5Dcreate_simple.vi"("ndims"=1, "error in (no error)"=w9, "type in"=w8, "name"=w3, "ref in"=w2) -> ("dset out"=w7:T15)  [unwired: 5 in, 1 out]
  n6 = for {
    N: 4 -> [_]
    tunnel: w7 -> [w22]
    tunnel: [w20] -> w6
    tunnel: [w21] -> w5
    tunnel: w3 -> [w19]
    w43 = T1 {"Timestring"="", "Timestamp"=0.0, "MaxValue"=0.0, "PeakLoc"=0.0, "df"=0.0}  # HDF5_ToneInfo
    # "Write Cal info"
    # "Convert to a cluster that HDF5 can use:\nNamed elements keep their name and attributes.\nNo array within the cluster"
    n7 = Get Date/Time In Seconds() -> (seconds since 1Jan1904=w31:timestamp)
    n8 = Wait (ms)(milliseconds to wait=u32 1000) -> ()  [unwired: 1 out]
    n9 = Get Date/Time String(seconds (now)=w31, want seconds? (F)=TRUE) -> (date string=w34:string, time string=w33:string)  [unwired: 1 in]
    n10 = Increment(x=TargetNumber."1" ("input 1")) -> (x+1=w24:T13)
    n11 = Concatenate Strings(w34, w33) -> (w32:string)
    n12 = Format Into String(format string="Tone%d", w24) -> (resulting string=w26:string)  [unwired: 2 in, 1 out]
    n13 = Bundle By Name(cluster=w43, "Timestring"=w32, "Timestamp"=w31, "MaxValue"=1.1, "PeakLoc"=2.2 ("MaxValue"), "df"=3.3 ("MaxValue")) -> (w29:T1)
    n14 = call <vilib>:"H5Dappend.vi"("create? (T)"=TRUE, "data"=w29, "ref in"=w22) -> ("error out"=w18:errorcluster, "ref out"=w20:T15)  [unwired: 5 in, 2 out]
    n15 = Unbundle By Name(T50 {"LastPk"=0.0, "Shift_"=-24999462.633451957, "Pk_PreShift"=0.0, "Peak_ToFPGA"=-24999462.633451957, "MaxValue"=0.0, "MaxIndex"=0, "Tone"={"PeakLoc"=0.0, "df_"=0.0, "ZoomPwr"=[0.0, 0.0, 0.0, 0.0, 0.0, 0.0, 0.0, 0.0, 8.8, 9.9, 10.1], "ZoomPhase"=[]}, "TimeDomainI"=array[12500 elements], "TimeDomainQ"=[], "PwrSpectrum"=[], "RunningAvgFreq"=0.0, "PhaseSpect"=[], "RealSpect"=[], "ImagSpect"=[]} ("input cluster")) -> ("Tone.ZoomPwr"=w28:dbl[])
    n16 = disable-structure shown="Enabled" {
      disable-tunnel: [w54 w56] -> w42
      disable-tunnel: [w50 w55] -> w30
      disable-tunnel: w28 -> [w49 _]
      disable-tunnel: w20 -> [w47 w56]
      disable-tunnel: w19 -> [w46 _]
      disable-tunnel: w18 -> [w45 w55]
      frame Disabled {
        # "Write Cal Zoom"
        n17 = call <vilib>:"H5Gopen.vi"("create? (F)"=TRUE, "error in (no error)"=w45, "name"="Zoom", "ref in"=w47) -> ("group out"=w51:T15)  [unwired: 6 in, 1 out]
        n18 = call <vilib>:"H5Dappend.vi"("create? (T)"=TRUE, "dataset name"=w46, "data"=w49, "ref in"=w51) -> ("error out"=w50:errorcluster, "ref out"=w54:T15)  [unwired: 4 in, 2 out]
      }
      frame Enabled {
      }
    }
    n19 = disable-structure shown="Enabled" {
      disable-tunnel: w30 -> [w67 w73]
      disable-tunnel: w29 -> [w66 _]
      disable-tunnel: w28 -> [w62 _]
      disable-tunnel: [w61 w73] -> w27
      disable-tunnel: w26 -> [w60 _]
      disable-tunnel: w22 -> [w57 _]
      frame Disabled {
        # "Write Beac Zoom"
        # "Write Beac info"
        n20 = Concatenate Strings(w60, "\\Beac" ("string")) -> (w70:string)
        n21 = call <vilib>:"H5Gopen.vi"("create? (F)"=TRUE, "error in (no error)"=w67, "name"=w70, "ref in"=w57) -> ("group out"=w68:T15)  [unwired: 6 in, 1 out]
        n22 = call <vilib>:"H5Dappend.vi"("create? (T)"=TRUE, "dataset name"=w60, "data"=w66, "ref in"=w68) -> ("ref out"=w65:T15)  [unwired: 4 in, 3 out]
        n23 = call <vilib>:"H5Gopen.vi"("create? (F)"=TRUE, "name"="Zoom", "ref in"=w65) -> ("group out"=w63:T15)  [unwired: 7 in, 1 out]
        n24 = call <vilib>:"H5Dappend.vi"("create? (T)"=TRUE, "dataset name"=w60, "data"=w62, "ref in"=w63) -> ("error out"=w61:errorcluster)  [unwired: 4 in, 3 out]
      }
      frame Enabled {
      }
    }
    n25 = xnode "H5Awrite.xnode"("error in (no error)"=w27, "data"=w32, "attrib name"="Timestamp" ("delimiter (Tab)"), "ref in"=w42) -> ("error out"=w21:errorcluster)  [unwired: 3 in, 2 out]
  }
  n26 = call <vilib>:"H5Dclose.vi"("error in (no error)"=w5, "dset in"=w6) -> ("error out"=w4:errorcluster)  [unwired: 9 in]
  n27 = call <vilib>:"H5Fclose.vi"("error in (no error)"=w4, "ref"=w2) -> ()  [unwired: 9 in, 1 out]
